vi "Module Top Level.vi"(8 "error in":errorcluster) -> (0 "error out":errorcluster)   [LabVIEW 2018, in "Testing UI 2.lvlib"]
doc: "This is the top level VI for this module. It uses a queue for communications and is stopped user a user event. The general architecture is similar to a simple queued message handler.\n\nThe VIs associated with this module are organized in a LabVIEW Library."
uses:
  Testing UI 2.lvlib
  Top Level/Shared Controls/All Data Cluster.ctl
  Top Level/Shared Controls/Acq Data.ctl
  Private Controls/UI  2 Data.ctl
  Private Controls/Module Data.ctl
  Private Controls/Module Action.ctl
  Top Level/Shared Controls/Range Updater.ctl
  Top Level/Shared Controls/APU Setup File.ctl
  Globals/Host Globals.vi
  Error Handler/Error Handler.lvlib
panel:
  in  "ARINC":bool
  in  "Main":bool
  in  "Calculated":bool
  in  "Accel Test":bool
  in  "EICAS":bool
  in  "Calibration":bool
  in  "Tab Control":T1(tab)
  out "TEUG4":dbl format="%.1f F"
  out "TUEG3":dbl format="%.1f F"
  out "TUEG2":dbl format="%.1f F"
  out "TUEG1":dbl format="%.1f F"
  out "TPO8":dbl format="%.1f F"
  out "TPO7":dbl format="%.1f F"
  out "TPO6":dbl format="%.1f F"
  out "TPO5":dbl format="%.1f F"
  out "TPO4":dbl format="%.1f F"
  out "TPO3":dbl format="%.1f F"
  out "TPO2":dbl format="%.1f F"
  out "TPO1":dbl format="%.1f F"
  out "TBAD4":dbl format="%.1f F"
  out "TBAD3":dbl format="%.1f F"
  out "TBAD2":dbl format="%.1f F"
  out "TBAD1":dbl format="%.1f F"
  out "TPI16":dbl format="%.1f F"
  out "TPI15":dbl format="%.1f F"
  out "TPI14":dbl format="%.1f F"
  out "TPI13":dbl format="%.1f F"
  out "TPI12":dbl format="%.1f F"
  out "TPI11":dbl format="%.1f F"
  out "TPI10":dbl format="%.1f F"
  out "TPI9":dbl format="%.1f F"
  out "TPI8":dbl format="%.1f F"
  out "TPI7":dbl format="%.1f F"
  out "TPI6":dbl format="%.1f F"
  out "TPI5":dbl format="%.1f F"
  out "TPI4":dbl format="%.1f F"
  out "TPI3":dbl format="%.1f F"
  out "TPI2":dbl format="%.1f F"
  out "TPI1":dbl format="%.1f F"
  out "00.00.9220.07":dbl(knob) caption="PAG-LO" scale=-50.0..150.0
  in  "00.00.9220.07":string
  out "C.38":dbl caption="TUEG Low" format="%.1f F"
  out "C.37":dbl caption="TUEG Up" format="%.1f F"
  out "C.12":cluster{dbl, dbl, dbl, dbl}(slide)={0.0, 380.23952095808386, 305.38922155688624, 392.21556886227546} caption="TEGTAVG" scale=400.0..1900.0
  out "C.12":dbl(slide) scale=400.0..1900.0
  in  "C.12":string
  out "C.25":cluster{dbl, dbl, dbl, dbl}(slide)={0.0, 380.23952095808386, 305.38922155688624, 392.21556886227546} caption="TEGT corr" scale=400.0..1900.0
  out "C.25":dbl(slide) scale=400.0..1900.0
  in  "C.25":string
  out "C.11":cluster{dbl, dbl, dbl, dbl}(slide)={0.0, 380.23952095808386, 305.38922155688624, 392.21556886227546} caption="TT1AVG" scale=0.0..150.0
  out "C.11":dbl(slide) scale=0.0..150.0
  in  "C.11":string
  out "C.02":cluster{dbl, dbl, dbl, dbl}(slide)={0.0, 380.23952095808386, 305.38922155688624, 392.21556886227546} caption="TEGT Meas" scale=400.0..1900.0
  out "C.02":dbl(slide) scale=400.0..1900.0
  in  "C.02":string
  out "C.32":dbl format="%.2f"
  out "C.31":dbl format="%.2f"
  out "00.03.9402":cluster{dbl, dbl}(knob)={0.0, 5.1101000456314445} caption="N1" scale=0.0..40640.0 scale format="%#.2f"
  out "C.17":dbl caption="MDOT" format="%.1f"
  out "C.18":dbl caption="Theta B" format="%.1f"
  out "C.19":dbl caption="PBmeas" format="%.1f"
  out "C.20":dbl caption="PBCOR" format="%.1f"
  out "C.21":dbl caption="Delta B" format="%.1f"
  out "C.22":dbl caption="Delta PAMB" format="%.1f"
  out "02.03.9227.00":dbl(knob) caption="SVTMC" scale=0.0..120.0
  out "C.29":dbl caption="HPkw" format="%.1f"
  out "02.04.9871.12":dbl caption="TkVA" format="%.1f"
  out "02.04.9871.13":dbl caption="Freq" format="%.1f"
  out "C.51":cluster{dbl, dbl, dbl, dbl}(slide)={0.0, 380.23952095808386, 305.38922155688624, 392.21556886227546} caption="Tamb" scale=55.0..125.0
  out "C.51":dbl(slide) caption="DCF" scale=55.0..125.0
  in  "C.51":string
  in  "01.01.9213.12":string
  in  "01.01.9213.13":string
  in  "01.01.9213.14":string
  in  "01.01.9213.15":string
  in  "01.01.9213.00":string
  in  "01.01.9213.01":string
  in  "01.01.9213.02":string
  in  "01.01.9213.03":string
  out "00.00.9220.12":dbl(knob) caption="PBA660" scale=0.0..50.0
  in  "00.00.9220.12":string
  out "00.00.9220.14":dbl(knob) caption="PBA290" scale=0.0..50.0
  in  "00.00.9220.14":string
  out "00.00.9220.15":dbl(knob) caption="PBA300" scale=0.0..50.0
  in  "00.00.9220.15":string
  out "00.00.9220.11":dbl(knob) caption="PES" scale=-50.0..150.0
  in  "00.00.9220.11":string
  out "00.00.9220.02":dbl(knob) caption="PFI" scale=0.0..100.0
  in  "00.00.9220.02":string
  out "00.00.9220.01":dbl(knob) caption="PFPD" scale=0.0..600.0
  in  "00.00.9220.01":string
  out "00.00.9220.03":dbl(knob) caption="POPD" scale=0.0..200.0
  in  "00.00.9220.03":string
  out "00.00.9220.08":dbl(knob) caption="PAG-HI" scale=-30.0..15.0
  in  "00.00.9220.08":string
  out "00.00.9220.09":dbl(knob) caption="PTBC" scale=-50.0..150.0
  in  "00.00.9220.09":string
  out "C.52":dbl(knob) caption="PBAD" scale=0.0..120.0
  in  "C.52":string
  out "C.49":cluster{dbl, dbl}(knob)={0.0, 94.00905280256501} caption="WBmeas"
  in  "C.49":string
  out "01.00.9213.11":cluster{dbl, dbl, dbl, dbl}(slide)={0.0, 380.23952095808386, 305.38922155688624, 392.21556886227546} caption="Tamb" scale=0.0..150.0 scale format="%.2f F"
  out "01.00.9213.11":dbl(slide) caption="TAMB" scale=0.0..150.0
  in  "01.00.9213.11":string
  out "00.00.9220.04":cluster{dbl, dbl, dbl, dbl}(slide)={0.0, 380.23952095808386, 305.38922155688624, 392.21556886227546} caption="Tamb" scale=0.0..31.0 scale format="%.2f"
  out "00.00.9220.04":dbl(slide) caption="PBAR" scale=0.0..31.0
  in  "00.00.9220.04":string
  out "C.53":cluster{dbl, dbl, dbl, dbl}(slide)={0.0, 380.23952095808386, 305.38922155688624, 392.21556886227546} caption="Tamb" scale=0.0..100.0
  out "C.53":dbl(slide) caption="POI" scale=0.0..100.0
  in  "C.53":string
  out "00.00.9220.06":cluster{dbl, dbl, dbl, dbl}(slide)={0.0, 380.23952095808386, 305.38922155688624, 392.21556886227546} caption="Tamb" scale=0.0..300.0 scale format="%.2f"
  out "00.00.9220.06":dbl(slide) caption="POD" scale=0.0..300.0
  in  "00.00.9220.06":string
  out "01.00.9213.04":cluster{dbl, dbl, dbl, dbl}(slide)={0.0, 380.23952095808386, 305.38922155688624, 392.21556886227546} caption="Tamb" scale=0.0..600.0 scale format="%.1f F"
  out "01.00.9213.04":dbl(slide) caption="TOI" scale=0.0..600.0
  in  "01.00.9213.04":string
  out "01.00.9213.07":cluster{dbl, dbl, dbl, dbl}(slide)={0.0, 380.23952095808386, 305.38922155688624, 392.21556886227546} caption="TFPI" scale=0.0..150.0
  out "01.00.9213.07":dbl(slide) scale=0.0..150.0
  out "01.00.9213.10":cluster{dbl, dbl, dbl, dbl}(slide)={0.0, 380.23952095808386, 305.38922155688624, 392.21556886227546} caption="TFC" scale=0.0..200.0
  out "01.00.9213.10":dbl(slide) scale=0.0..200.0
  in  "01.00.9213.10":string
  out "01.00.9213.02":cluster{dbl, dbl, dbl, dbl}(slide)={0.0, 380.23952095808386, 305.38922155688624, 392.21556886227546} caption="TOPD" scale=0.0..300.0
  out "01.00.9213.02":dbl(slide) scale=0.0..300.0
  out "01.00.9213.09":cluster{dbl, dbl, dbl, dbl}(slide)={0.0, 380.23952095808386, 305.38922155688624, 392.21556886227546} caption="TFFT" scale=0.0..200.0
  out "01.00.9213.09":dbl(slide) scale=0.0..200.0
  out "01.00.9213.08":cluster{dbl, dbl, dbl, dbl}(slide)={0.0, 380.23952095808386, 305.38922155688624, 392.21556886227546} caption="TLCI" scale=0.0..150.0
  out "01.00.9213.08":dbl(slide) scale=0.0..150.0
  out "01.00.9213.06":cluster{dbl, dbl, dbl, dbl}(slide)={0.0, 380.23952095808386, 305.38922155688624, 392.21556886227546} caption="TCD" scale=0.0..600.0
  out "01.00.9213.06":dbl(slide) scale=0.0..600.0
  out "TUEG Delta":dbl caption="Delta" format="%.1f F"
  out "02.04.9871.00":dbl caption="L1V" format="%.1f"
  out "02.04.9871.01":dbl caption="L2V" format="%.1f"
  out "02.04.9871.02":dbl caption="L3V" format="%.1f"
  out "02.04.9871.09":dbl caption="L1A" format="%.1f"
  out "02.04.9871.10":dbl caption="L2A" format="%.1f"
  out "02.04.9871.11":dbl caption="L3A" format="%.1f"
  out "02.04.9871.03":dbl caption="L2L1V" format="%.1f"
  out "02.04.9871.04":dbl caption="L3L2V" format="%.1f"
  out "02.04.9871.05":dbl caption="L1L3V" format="%.1f"
  out "02.04.9871.06":dbl caption="L1NV" format="%.1f"
  out "02.04.9871.07":dbl caption="L2NV" format="%.1f"
  out "02.04.9871.08":dbl caption="L3NV" format="%.1f"
  out "02.04.9871.14":dbl caption="Power" format="%.1f"
  out "RH":dbl(slide)
  in  "RH":string
  in  "02.02.9402":string
  in  "01.01.9213.07":string
  in  "01.01.9213.06":string
  in  "01.01.9213.05":string
  in  "01.01.9213.04":string
  in  "01.01.9213.11":string
  in  "01.01.9213.10":string
  in  "01.01.9213.09":string
  in  "01.01.9213.08":string
  out "C.30":cluster{dbl, dbl, dbl, dbl}(slide)={0.0, 380.23952095808386, 305.38922155688624, 392.21556886227546} caption="TBmeas" scale=0.0..600.0
  out "C.30":dbl(slide) scale=0.0..600.0
  in  "C.30":string
  out "00.00.9220.03":dbl caption="POPD"
  out "C.02":dbl caption="TEGT Meas"
  out "EGT Measured and Oil Pressure":T2(graph)
  out "C.32":dbl caption="N2 %" format="%.1f %"
  out "C.31":dbl caption="N1 %" format="%.1f %"
  out "00.03.9402":cluster{dbl, dbl}(knob)={0.0, 5.1101000456314445} scale=0.0..40400.0
  out "C.39":dbl caption="OrifDia"
  out "C.26":dbl caption="K"
  out "C.01":dbl caption="SG60"
  out "C.00":dbl caption="AIN" format="%#_g ft^2"
  out "02.03.9227.02":dbl(knob) caption="EICAS EGT" scale=0.0..2000.0
  out "02.03.9227.01":dbl(knob) caption="ECU N2" scale=0.0..40400.0
  out "CaliData":T3 caption="All Data Cluster"
  out "RawData":T3 caption="All Data Cluster"
  out "ARINCValues":string[](array[string])
  out "ARINCLabels":string[][](array[string])
  # "Enviromental Conditions"
  # "Cell Orifice Conditions"
  # "APU Bleed Air"
  # "APU INLET"
  # "TC splits"
  # "Rotor Speed"
  # "APU Fluids Status"
  # "APU EXHAUST"
  # "N1"
  # "N2"
  # "N1%"
  # "N2%"
  # "APU UNIT EXHAUST"
  # "APU Buffered Air Pressures"
  # "Standard Corrections"
  # "APU MISC"
  # "BLEED"
  # "Bleed"
  # "Day"
  # "APU Temperatures"
  # "Power"
  # "Load Bank"
  # "Acceleration Test"
  # "Rotor Speed"
  # "Default:  42000       2000      100"
  # "N1"
  # "N1"
  # "Calculated"
  # "User Inputs:"
  # "A \nA = K(2*gc/R)^0.5"
  # "P1\nPOIab * 70.726"
  # "PB meas P  (PSI)\n\nPBADab*(0.491154)"
  # "HPkw\nPower *1.34102209"
  # "SGII\nSG60*(1+(0.003688+-0.006518*SG60+0.003194*SG60^2)*(60-TFFT));"
  # "PODF\nPOD * 5.2"
  # "B \nB = Y1(1-(P2/P1))0.5 ="
  # "RhoFuel\n-0.0249876*TFFT + 52.2080853"
  # "PBCOR\n((PBMEAS P) / ((Pbar*0.491154)/14.7))"
  # "P2\nP1-PODF"
  # "RhoH2O\n0.000000162*TFFT^3 - 0.000127783*TFFT^2 + 0.008195247*TFFT + 62.294045686"
  # "C \nC = (TOI)^0.5/P1*A\nTOI to Rankeine for calculation"
  # "DeltaB\n((PBMeas P))/14.7;"
  # "P1P2\nP1-P2"
  # "SGCal\nRhoFuel / RhoH2O"
  # "dPAMB\n(PBAR * 0.491154)/(14.7/))"
  # "WBmeas \n(A*B)/C"
  # "RP1P2\n(P1-P2)/P1"
  # "Rho_air\n(PSAVG *144)/ 53.35*(TPIAVG + 459.67)"
  # "Pamb P\n(PBAR*0.491154)"
  # "WBcor \nWBCOR = WBMEAS/dPAMB"
  # "VIN\n(2/Rho_air)*(PDAVG - PSAVG)^ 1/2"
  # "Y1\n\n3.025\n=-0.2991*RP1P2 + 1.0006\n\n4\n=-0.305*RP1P2 + 1.0008\n\n5\n=-0.3.18*RP1P2 + 1.001"
  # "DPPb\n[14.7*(PBMEAS P+ PBAR)/(PBAR)]-14.7"
  # "MDOT\nMDOT = Rho_air * AIN * VIN"
  # "DCF \nWBmeas*((qB)^0.5)/DeltaB"
  # "TEGTcorr\nTEGTMeas - 11 (PBCOR-PBCOR-from-table)"
  # "ThetaB\n(TBMEAS + 459.7)/518.7"
  # "FlowPPH\n= Flow(GPH)*60*RhoFuel/7.48"
  # "EICAS"
  # "Description"
  # "Units"
  # "Value"
  # "Label"
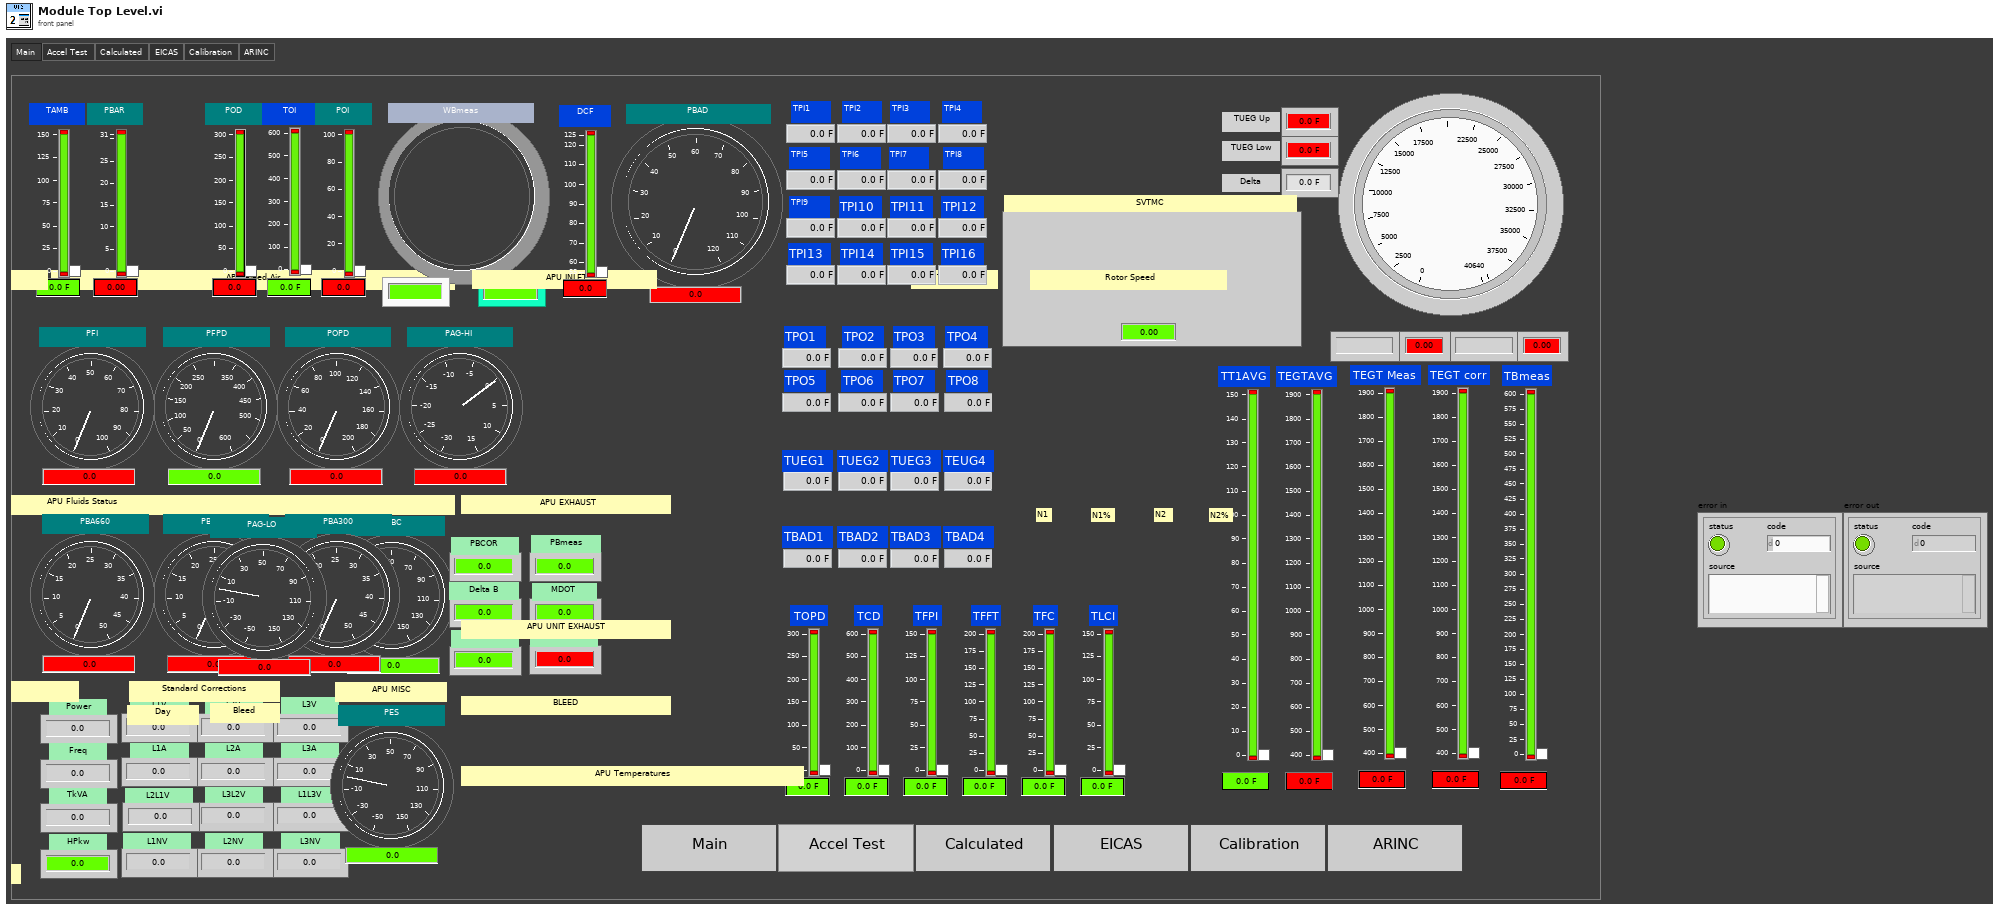
[diagram p1: front panel]
types:
  T1 = enum32{"Main", "Accel Test", "Calculated", "EICAS", "Calibration", "ARINC"}
  T2 = cluster{"RPM":dbl, "TEGT ":dbl, "Oil Pressure":dbl}
  T3 = typedef "All Data Cluster.ctl" = cluster{"AI":T4, "Accel Data":cluster{"Accel RMS(in/sec2)":dbl[], "Accel Peak(in/sec2)":dbl[], "Velocity RMS(in/sec)":dbl[], "Velocity Peak(in/sec)":dbl[]}, "Temps":cluster{"01-00-9213":dbl[], "01-01-9213":dbl[], "01-02-9213":dbl[]}, "00-03-9402(RPM)":dbl[], "02-04-9871":dbl[], "ARINC":sgl[]}
  T4 = typedef "Acq Data.ctl" = cluster{"00-00-9220":dbl[], "00-01-9220":dbl[], "02-02-9219":dbl[], "02-03-9227":dbl[], "02-05-9205":dbl[]}
  T5 = typedef "Testing UI 2.lvlib/UI  2 Data.ctl" = cluster{"[Array Of Threshold Refs]":refnum<vi>[], "[Slider Indicator Refs]":refnum<vi>[], "[Knob Indicator Refs]":refnum<vi>[], "[Digital Indicator Refs]":refnum<vi>[], "[Digital Temp]":refnum<vi>[]}
  T6 = enum32{"Main", "Accel Test", "Calculated", "EICAS", "Calibration"}
  T7 = enum32{"Invalid", "Standard", "Closed", "Hidden", "Minimized", "Maximized"}
  T8 = typedef "APU Setup File.ctl" = cluster{"Sensor Info":string[][], "Variables":string[][], "CMM Table 106":string[][], "CMM Table 106B ":string[][], "Accel Config":string[][], "Report Sheet 1":string[][], "Report Sheet 2":string[][], "Report Sheet 3":string[][]}
  T9 = typedef "Range Updater.ctl" = cluster{"[Digital Indicator Refs]":refnum<vi>[], "[Knob Indicator Refs]":refnum<vi>[], "[Slider Indicator Refs]":refnum<vi>[], "[Bool Indicator Refs]":refnum<vi>[], "[[Sensor Info]]":string[][], "[Array Of Threshold Refs]":refnum<vi>[]}
  T10 = typedef "Testing UI 2.lvlib/Module Data.ctl" = cluster{"Data":variant, "Action":T11}
  T11 = typedef "Testing UI 2.lvlib/Module Action.ctl" = enum8{"Init", "Open FP", "Error", "Exit", "Timeout", "Load APU Setup"}
  T12 = typedef "Calculated Data.ctl" = cluster{"C.00":dbl, "C.01":dbl, "C.02":dbl, "C.03":dbl, "C.04":dbl, "C.05":dbl, "C.06":dbl, "C.07":dbl, "C.08":dbl, "C.09":dbl, "C.10":dbl, "C.11":dbl, "C.12":dbl, "C.13":dbl, "C.14":dbl, "C.15":dbl, "C.16":dbl, "C.17":dbl, "C.18":dbl, "C.19":dbl, "C.20":dbl, "C.21":dbl, "C.22":dbl, "C.23":dbl, "C.24":dbl, "C.25":dbl, "C.26":dbl, "C.27":dbl, "C.28":dbl, "C.29":dbl, "C.30":dbl, "C.31":dbl, "C.32":dbl, "C.33":dbl, "C.34":dbl, "C.35":dbl, "C.36":dbl, "C.37":dbl, "C.38":dbl, "C.39":dbl, "C.40":dbl, "C.41":dbl, "C.42":dbl, "C.43":dbl, "C.44":dbl, "C.45":dbl, "C.46":dbl, "C.47":dbl, "C.48":dbl, "C.49":dbl, "C.50":dbl, "C.51":dbl, "C.52":dbl, "C.53":dbl, "C.54":dbl, "C.55":dbl, "C.56":dbl, "C.57":dbl, "C.58":dbl, "C.59":dbl, "C.60":dbl, "C.61":dbl, "C.62":dbl}
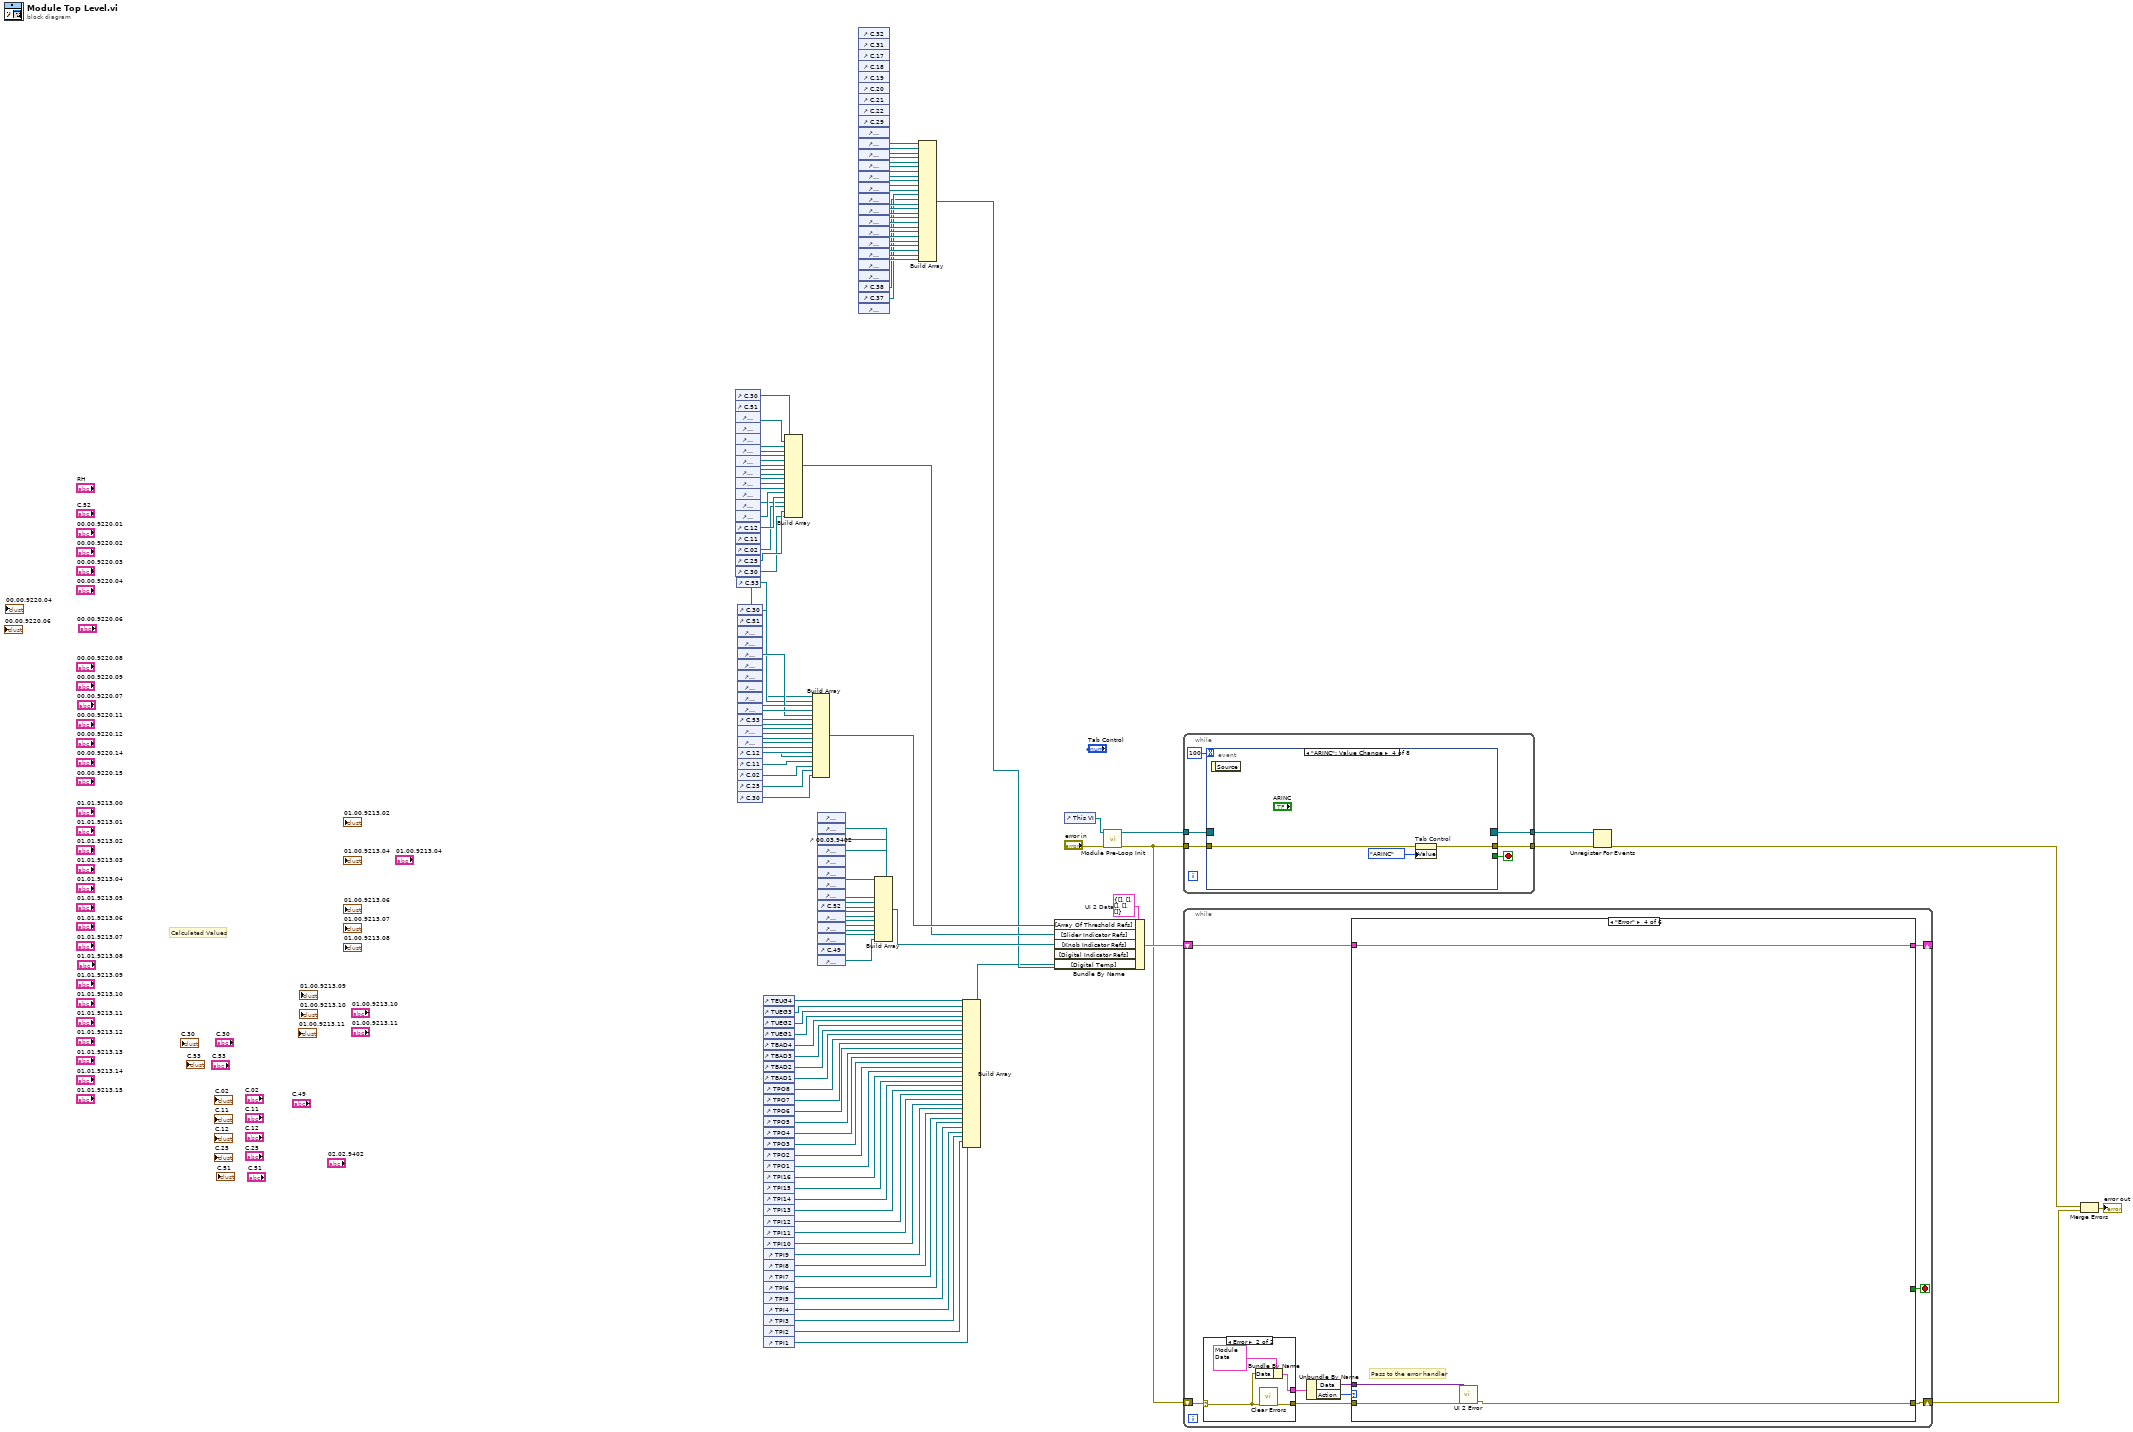
[diagram p0: block diagram]
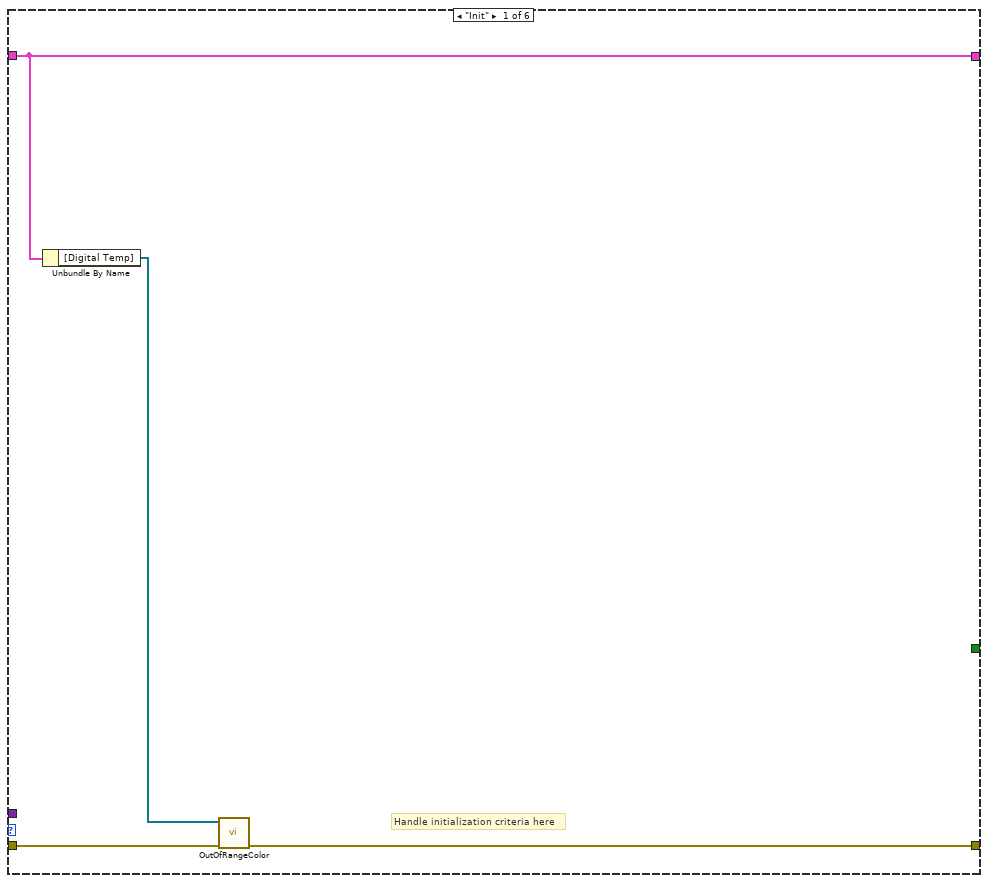
[diagram p2: hidden frame]
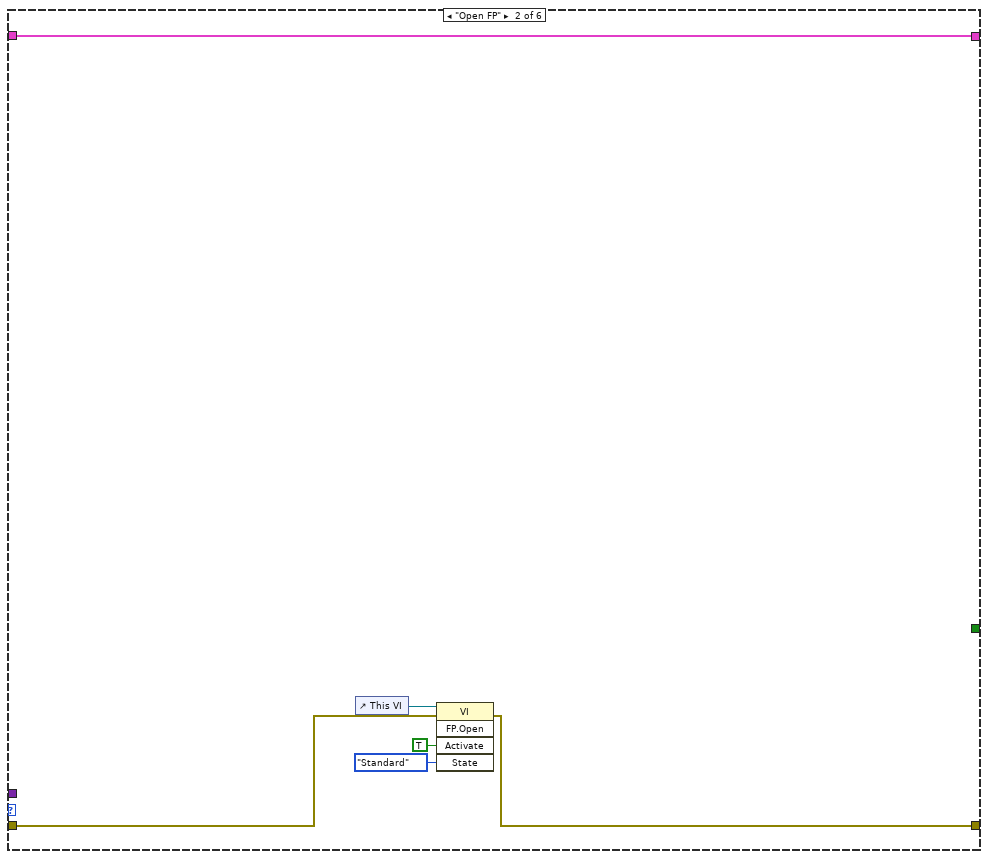
[diagram p3: hidden frame]
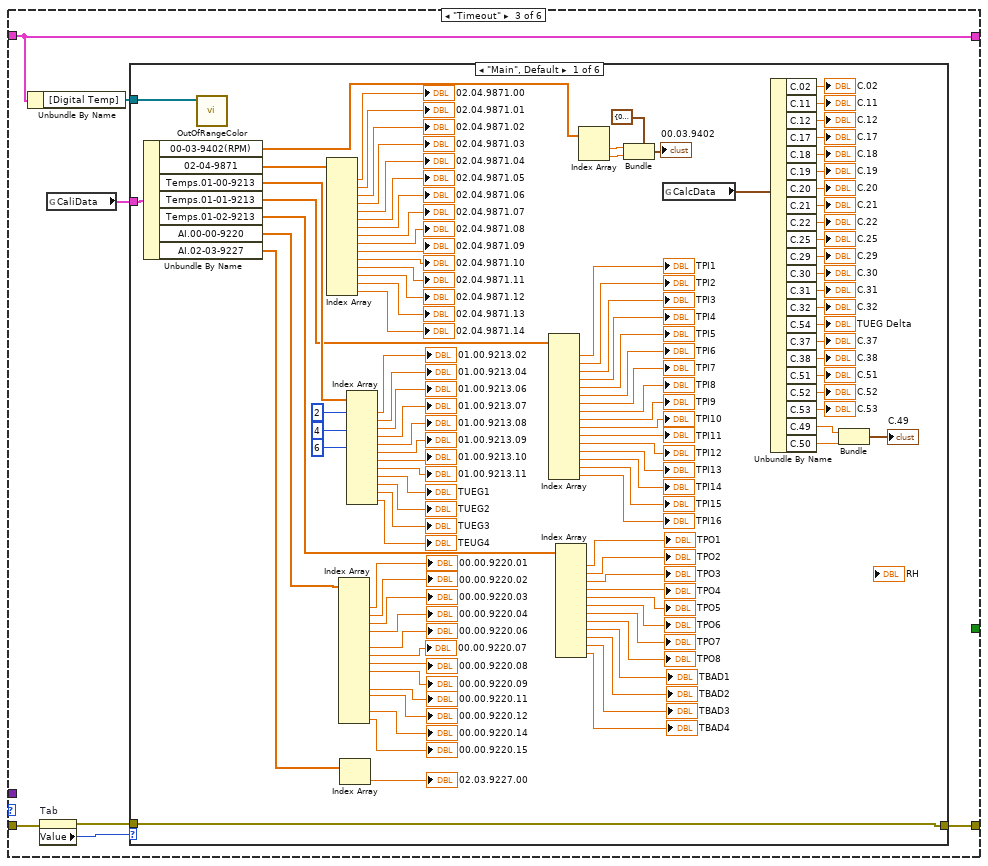
[diagram p4: hidden frame]
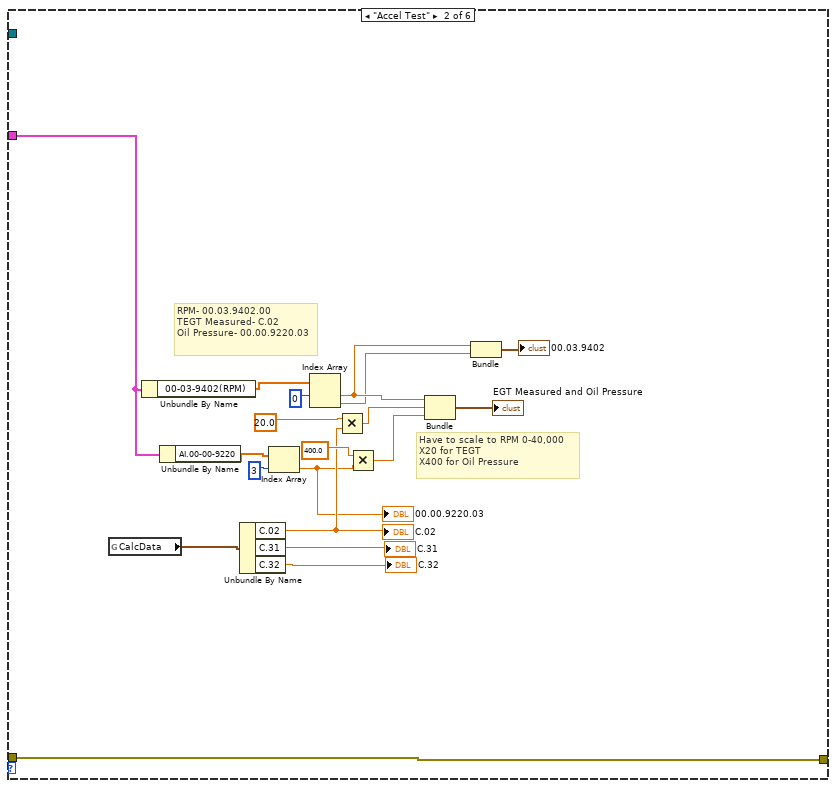
[diagram p5: hidden frame]
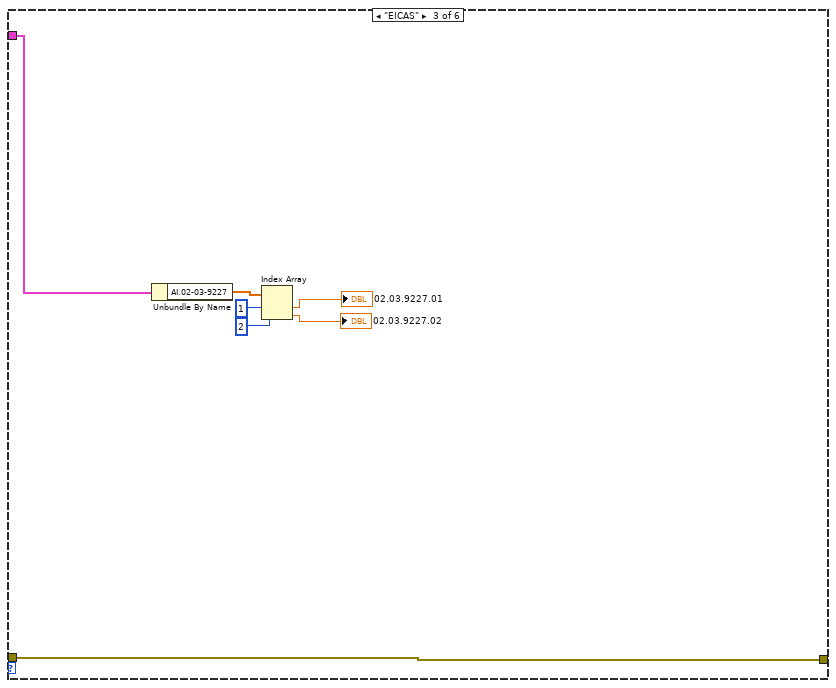
[diagram p6: hidden frame]
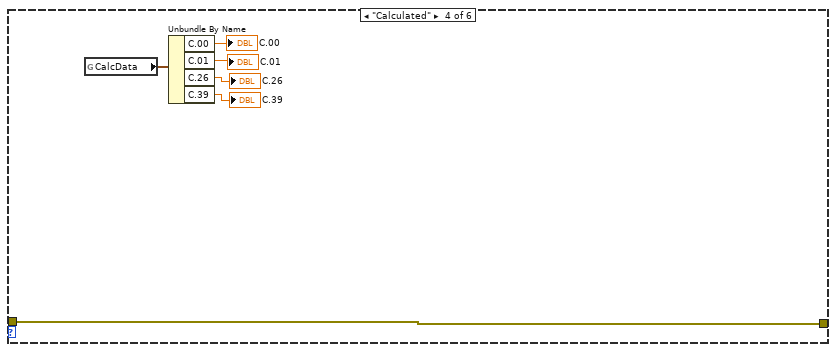
[diagram p7: hidden frame]
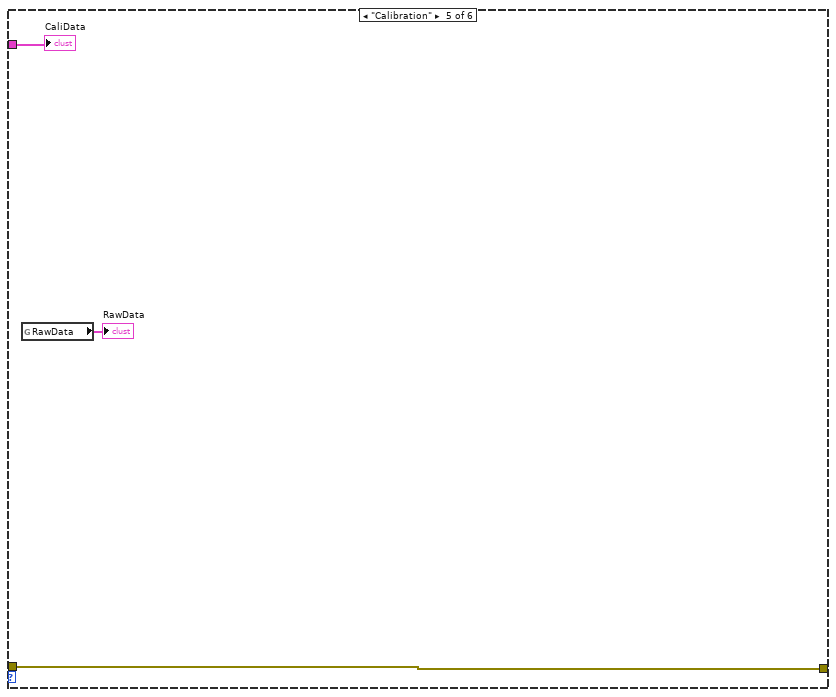
[diagram p8: hidden frame]
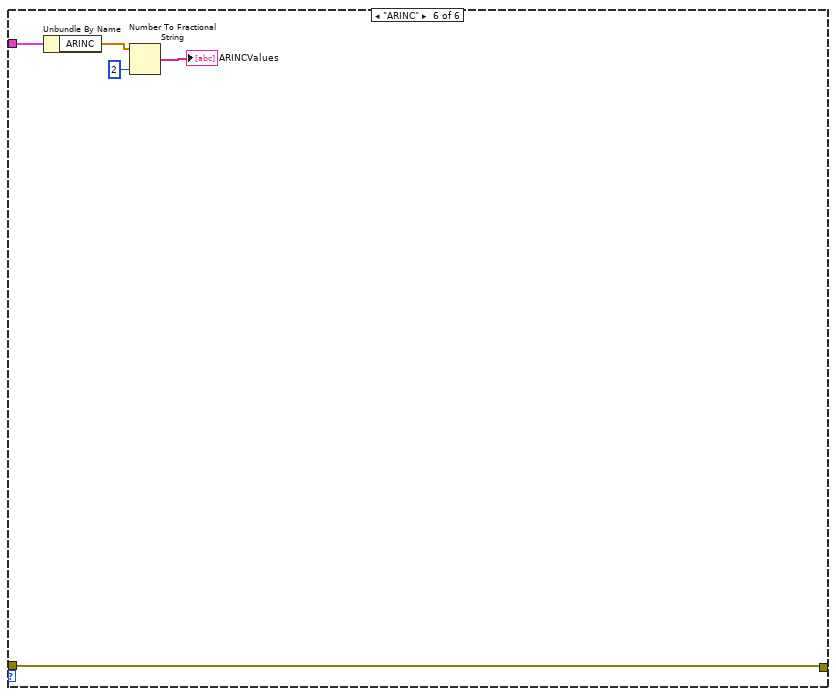
[diagram p9: hidden frame]
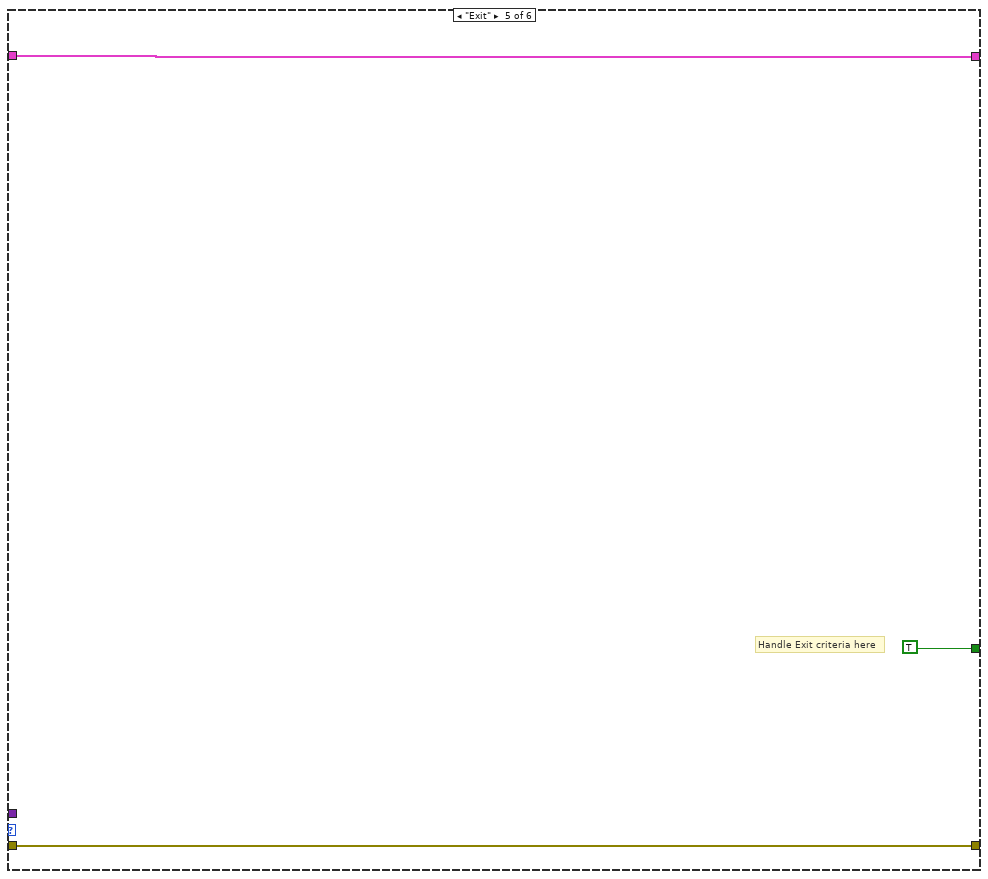
[diagram p10: hidden frame]
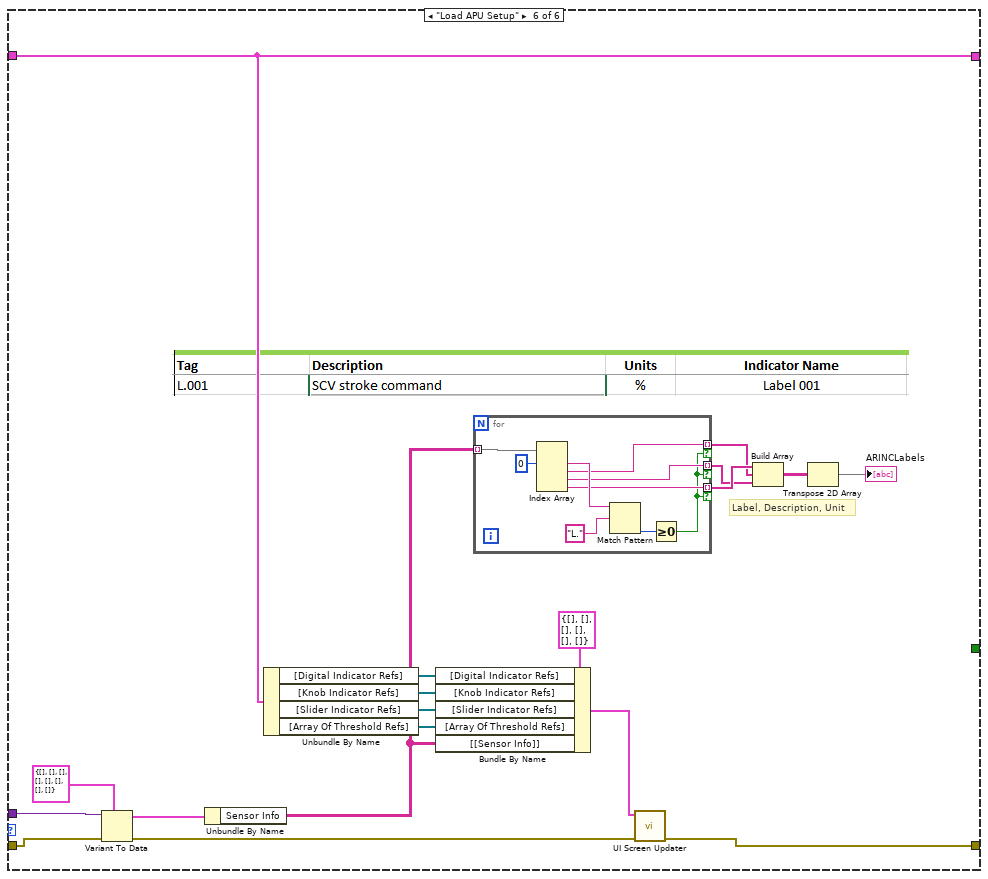
[diagram p11: hidden frame]
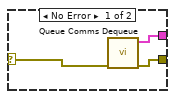
[diagram p12: hidden frame]
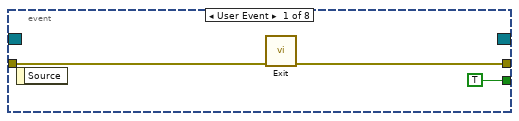
[diagram p13: hidden frame]
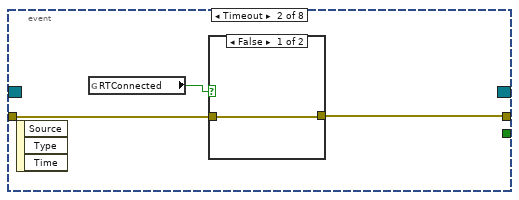
[diagram p14: hidden frame]
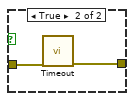
[diagram p15: hidden frame]
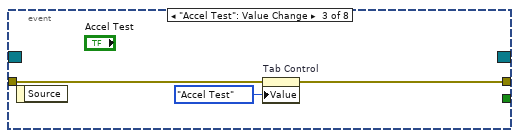
[diagram p16: hidden frame]
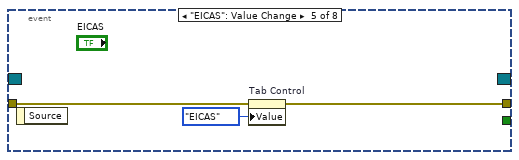
[diagram p17: hidden frame]
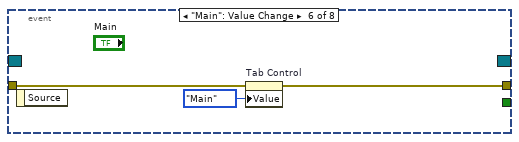
[diagram p18: hidden frame]
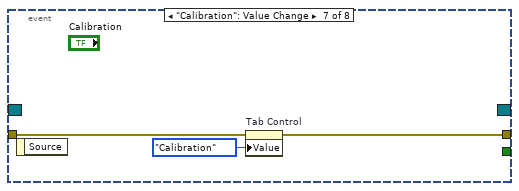
[diagram p19: hidden frame]
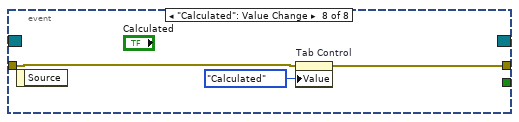
[diagram p20: hidden frame]
diagram:
  w116 = T5 {"[Array Of Threshold Refs]"=[], "[Slider Indicator Refs]"=[], "[Knob Indicator Refs]"=[], "[Digital Indicator Refs]"=[], "[Digital Temp]"=[]}  # UI 2 Data
  # "Calculated Values"
  n1 = control-ref of="C.30"() -> (w37:refnum<vi>)
  n2 = control-ref of="C.51"() -> (w38:refnum<vi>)
  n3 = control-ref of="01.00.9213.06"() -> (w102:refnum<vi>)
  n4 = control-ref of="01.00.9213.08"() -> (w101:refnum<vi>)
  n5 = control-ref of="01.00.9213.09"() -> (w100:refnum<vi>)
  n6 = control-ref of="01.00.9213.02"() -> (w99:refnum<vi>)
  n7 = control-ref of="01.00.9213.10"() -> (w98:refnum<vi>)
  n8 = control-ref of="01.00.9213.07"() -> (w97:refnum<vi>)
  n9 = control-ref of="01.00.9213.04"() -> (w96:refnum<vi>)
  n10 = control-ref of="00.00.9220.06"() -> (w95:refnum<vi>)
  n11 = control-ref of="00.00.9220.04"() -> (w93:refnum<vi>)
  n12 = control-ref of="01.00.9213.11"() -> (w92:refnum<vi>)
  n13 = control-ref of="C.12"() -> (w45:refnum<vi>)
  n14 = control-ref of="C.11"() -> (w44:refnum<vi>)
  n15 = control-ref of="C.02"() -> (w3:refnum<vi>)
  n16 = control-ref of="C.25"() -> (w43:refnum<vi>)
  n17 = control-ref of="C.30"() -> (w42:refnum<vi>)
  n18 = control-ref of="C.53"() -> (w94:refnum<vi>)
  n19 = control-ref of="C.30"() -> (w35:refnum<vi>)
  n20 = control-ref of="C.51"() -> (w36:refnum<vi>)
  n21 = control-ref of="01.00.9213.06"() -> (w114:refnum<vi>)
  n22 = control-ref of="01.00.9213.08"() -> (w113:refnum<vi>)
  n23 = control-ref of="01.00.9213.09"() -> (w112:refnum<vi>)
  n24 = control-ref of="01.00.9213.02"() -> (w111:refnum<vi>)
  n25 = control-ref of="01.00.9213.10"() -> (w110:refnum<vi>)
  n26 = control-ref of="01.00.9213.07"() -> (w109:refnum<vi>)
  n27 = control-ref of="01.00.9213.04"() -> (w108:refnum<vi>)
  n28 = control-ref of="00.00.9220.06"() -> (w107:refnum<vi>)
  n29 = control-ref of="C.53"() -> (w106:refnum<vi>)
  n30 = control-ref of="00.00.9220.04"() -> (w105:refnum<vi>)
  n31 = control-ref of="01.00.9213.11"() -> (w104:refnum<vi>)
  n32 = control-ref of="C.12"() -> (w50:refnum<vi>)
  n33 = control-ref of="C.11"() -> (w49:refnum<vi>)
  n34 = control-ref of="C.02"() -> (w48:refnum<vi>)
  n35 = control-ref of="C.25"() -> (w47:refnum<vi>)
  n36 = control-ref of="C.30"() -> (w46:refnum<vi>)
  n37 = control-ref of="TEUG4"() -> (w34:refnum<vi>)
  n38 = control-ref of="TUEG3"() -> (w33:refnum<vi>)
  n39 = control-ref of="TUEG2"() -> (w32:refnum<vi>)
  n40 = control-ref of="TUEG1"() -> (w31:refnum<vi>)
  n41 = control-ref of="TBAD4"() -> (w30:refnum<vi>)
  n42 = control-ref of="TBAD3"() -> (w29:refnum<vi>)
  n43 = control-ref of="TBAD2"() -> (w28:refnum<vi>)
  n44 = control-ref of="TBAD1"() -> (w27:refnum<vi>)
  n45 = control-ref of="TPO8"() -> (w26:refnum<vi>)
  n46 = control-ref of="TPO7"() -> (w25:refnum<vi>)
  n47 = control-ref of="TPO6"() -> (w24:refnum<vi>)
  n48 = control-ref of="TPO5"() -> (w23:refnum<vi>)
  n49 = control-ref of="TPO4"() -> (w22:refnum<vi>)
  n50 = control-ref of="TPO3"() -> (w21:refnum<vi>)
  n51 = control-ref of="TPO2"() -> (w20:refnum<vi>)
  n52 = control-ref of="TPO1"() -> (w19:refnum<vi>)
  n53 = control-ref of="TPI16"() -> (w18:refnum<vi>)
  n54 = control-ref of="TPI15"() -> (w17:refnum<vi>)
  n55 = control-ref of="TPI14"() -> (w16:refnum<vi>)
  n56 = control-ref of="TPI13"() -> (w15:refnum<vi>)
  n57 = control-ref of="TPI12"() -> (w14:refnum<vi>)
  n58 = control-ref of="TPI11"() -> (w13:refnum<vi>)
  n59 = control-ref of="TPI10"() -> (w12:refnum<vi>)
  n60 = control-ref of="TPI9"() -> (w11:refnum<vi>)
  n61 = control-ref of="TPI8"() -> (w10:refnum<vi>)
  n62 = control-ref of="TPI7"() -> (w9:refnum<vi>)
  n63 = control-ref of="TPI6"() -> (w8:refnum<vi>)
  n64 = control-ref of="TPI5"() -> (w7:refnum<vi>)
  n65 = control-ref of="TPI4"() -> (w6:refnum<vi>)
  n66 = control-ref of="TPI3"() -> (w5:refnum<vi>)
  n67 = control-ref of="TPI2"() -> (w4:refnum<vi>)
  n68 = control-ref of="TPI1"() -> (w2:refnum<vi>)
  n69 = Build Array(w37, w38, w102, w101, w100, w99, w98, w97, w96, w95, w94, w93, w92, w45, w44, w3, w43, w42) -> (w91:refnum<vi>[])
  n70 = Build Array(w35, w36, w114, w113, w112, w111, w110, w109, w108, w107, w106, w105, w104, w50, w49, w48, w47, w46) -> (w103:refnum<vi>[])
  n71 = control-ref of="00.00.9220.15"() -> (w90:refnum<vi>)
  n72 = control-ref of="02.03.9227.00"() -> (w89:refnum<vi>)
  n73 = control-ref of="00.03.9402"() -> (w88:refnum<vi>)
  n74 = control-ref of="00.00.9220.12"() -> (w87:refnum<vi>)
  n75 = control-ref of="00.00.9220.01"() -> (w86:refnum<vi>)
  n76 = control-ref of="00.00.9220.03"() -> (w85:refnum<vi>)
  n77 = control-ref of="00.00.9220.09"() -> (w84:refnum<vi>)
  n78 = control-ref of="00.00.9220.14"() -> (w83:refnum<vi>)
  n79 = control-ref of="C.52"() -> (w82:refnum<vi>)
  n80 = control-ref of="00.00.9220.11"() -> (w81:refnum<vi>)
  n81 = control-ref of="00.00.9220.02"() -> (w80:refnum<vi>)
  n82 = control-ref of="00.00.9220.08"() -> (w79:refnum<vi>)
  n83 = control-ref of="C.49"() -> (w78:refnum<vi>)
  n84 = control-ref of="00.00.9220.07"() -> (w39:refnum<vi>)
  n85 = control-ref of="C.32"() -> (w77:refnum<vi>)
  n86 = control-ref of="C.31"() -> (w76:refnum<vi>)
  n87 = control-ref of="C.17"() -> (w75:refnum<vi>)
  n88 = control-ref of="C.18"() -> (w74:refnum<vi>)
  n89 = control-ref of="C.19"() -> (w73:refnum<vi>)
  n90 = control-ref of="C.20"() -> (w72:refnum<vi>)
  n91 = control-ref of="C.21"() -> (w71:refnum<vi>)
  n92 = control-ref of="C.22"() -> (w70:refnum<vi>)
  n93 = control-ref of="C.29"() -> (w69:refnum<vi>)
  n94 = control-ref of="02.04.9871.12"() -> (w68:refnum<vi>)
  n95 = control-ref of="02.04.9871.13"() -> (w67:refnum<vi>)
  n96 = control-ref of="02.04.9871.14"() -> (w66:refnum<vi>)
  n97 = control-ref of="02.04.9871.08"() -> (w65:refnum<vi>)
  n98 = control-ref of="02.04.9871.07"() -> (w64:refnum<vi>)
  n99 = control-ref of="02.04.9871.06"() -> (w63:refnum<vi>)
  n100 = control-ref of="02.04.9871.05"() -> (w62:refnum<vi>)
  n101 = control-ref of="02.04.9871.04"() -> (w61:refnum<vi>)
  n102 = control-ref of="02.04.9871.03"() -> (w60:refnum<vi>)
  n103 = control-ref of="02.04.9871.11"() -> (w59:refnum<vi>)
  n104 = control-ref of="02.04.9871.10"() -> (w58:refnum<vi>)
  n105 = control-ref of="02.04.9871.09"() -> (w57:refnum<vi>)
  n106 = control-ref of="02.04.9871.02"() -> (w56:refnum<vi>)
  n107 = control-ref of="02.04.9871.01"() -> (w55:refnum<vi>)
  n108 = control-ref of="C.38"() -> (w40:refnum<vi>)
  n109 = control-ref of="C.37"() -> (w41:refnum<vi>)
  n110 = control-ref of="02.04.9871.00"() -> (w54:refnum<vi>)
  n111 = Build Array(w90, w89, w88, w87, w86, w85, w84, w83, w82, w81, w80, w79, w78, w39) -> (w53:refnum<vi>[])
  n112 = Build Array(w77, w76, w75, w74, w73, w72, w71, w70, w69, w68, w67, w41, w40, w66, w65, w64, w63, w62, w61, w60, w59, w58, w57, w56, w55, w54) -> (w52:refnum<vi>[])
  n113 = Build Array(w34, w33, w32, w31, w30, w29, w28, w27, w26, w25, w24, w23, w22, w21, w20, w19, w18, w17, w16, w15, w14, w13, w12, w11, w10, w9, w8, w7, w6, w5, w4, w2) -> (w1:refnum<vi>[])
  n114 = Bundle By Name(cluster=w116, "[Array Of Threshold Refs]"=w103, "[Slider Indicator Refs]"=w91, "[Knob Indicator Refs]"=w53, "[Digital Indicator Refs]"=w52, "[Digital Temp]"=w1) -> (w115:T5)
  n115 = control-ref of="This VI"() -> (w124:refnum<vi>)
  n116 = call "Module Pre-Loop Init.vi"("error in (no error)"="error in", "Top Level VI Ref in"=w124) -> ("error out"=w51:errorcluster, "User Event Stop Ref"=w122:refnum<event-registration>)  [unwired: 8 in]
  n117 = while {
    tunnel: w122 -> [w130]
    tunnel: [w129] -> w120
    tunnel: w51 -> [w128]
    tunnel: [w126] -> w121
    stop <- w127 stop-if-true
    n118 = event shown="[3] \"ARINC\": Value Change" {
      selector: w130 -> [_ _ _ _ _ _ _ _]
      dyn-events: [_ _ _ _ _ _ _ _] -> w126
      timeout: 100 -> [_ _ _ _ _ _ _ _]
      tunnel: [w132 w135 w141 w143 w147 w150 w153 w156] -> w129
      tunnel: w128 -> [w131 w136 w142 w145 w148 w151 w154 w157]
      tunnel: [TRUE _ _ _ _ _ _ _] -> w127
      event User Event {
        n119 = event-data() -> ()  [unwired: 1 in, 1 out]
        n120 = call "Exit.vi"("error in"=w131) -> ("error out"=w132:errorcluster)  [unwired: 10 in]
      }
      event Timeout {
        n121 = event-data() -> ()  [unwired: 1 in, 3 out]
        n122 = global read "Host Globals.vi" "RTConnected"() -> (w134:bool)
        n123 = case shown="False" w134 {
          tunnel: w136 -> [w137 w139]
          tunnel: [w137 w138] -> w135
          frame False {
          }
          frame True {
            n124 = call "Timeout.vi"("error in (no error)"=w139) -> ("error out"=w138:errorcluster)  [unwired: 10 in]
          }
        }
      }
      event "Accel Test": Value Change {
        n125 = event-data() -> ()  [unwired: 1 in, 1 out]
        n126 = property on="Tab Control" class="TabCtl (strict)"(error in=w142, "Value"=T6."Accel Test" ("Tab Control")) -> (error out=w141:errorcluster)  [unwired: 1 in, 1 out]
      }
      event "ARINC": Value Change {
        n127 = event-data() -> ()  [unwired: 1 in, 1 out]
        n128 = property on="Tab Control" class="TabCtl (strict)"(error in=w145, "Value"=T1."ARINC" ("Tab Control")) -> (error out=w143:errorcluster)  [unwired: 1 in, 1 out]
      }
      event "EICAS": Value Change {
        n129 = event-data() -> ()  [unwired: 1 in, 1 out]
        n130 = property on="Tab Control" class="TabCtl (strict)"(error in=w148, "Value"=T6."EICAS" ("Tab Control")) -> (error out=w147:errorcluster)  [unwired: 1 in, 1 out]
      }
      event "Main": Value Change {
        n131 = event-data() -> ()  [unwired: 1 in, 1 out]
        n132 = property on="Tab Control" class="TabCtl (strict)"(error in=w151, "Value"=T6."Main" ("Tab Control")) -> (error out=w150:errorcluster)  [unwired: 1 in, 1 out]
      }
      event "Calibration": Value Change {
        n133 = event-data() -> ()  [unwired: 1 in, 1 out]
        n134 = property on="Tab Control" class="TabCtl (strict)"(error in=w154, "Value"=T6."Calibration" ("Tab Control")) -> (error out=w153:errorcluster)  [unwired: 1 in, 1 out]
      }
      event "Calculated": Value Change {
        n135 = event-data() -> ()  [unwired: 1 in, 1 out]
        n136 = property on="Tab Control" class="TabCtl (strict)"(error in=w157, "Value"=T6."Calculated" ("Tab Control")) -> (error out=w156:errorcluster)  [unwired: 1 in, 1 out]
      }
    }
  }
  n137 = while {
    shift-right: [w162] -> w119
    shift-left: w51 -> [w161]
    shift-right: [w160] -> _
    shift-left: w115 -> [w159]
    stop <- w158 stop-if-true
    n138 = case shown="Error" w161 {
      selector: w161 -> [w368 w371]
      tunnel: [w369 w372] -> w166
      tunnel: [w367 w370] -> w163
      frame No Error {
        n139 = call "Queue Comms Dequeue.vi"("error in (no error)"=w368) -> ("error out"=w367:errorcluster, "element"=w369:T10)  [unwired: 9 in]
      }
      frame Error {
        n140 = Bundle By Name(cluster=T10 {"Data"=variant, "Action"=enum."Error"} ("element"), "Data"=w371) -> (w372:T10)
        n141 = call <vilib>:"Clear Errors.vi"("error in (no error)"=w371) -> ("error out"=w370:errorcluster)  [unwired: 5 in, 1 out]
      }
    }
    n142 = Unbundle By Name(w166) -> ("Data"=w164:variant, "Action"=w165:T11)
    n143 = case shown="\"Error\"" w165 {
      tunnel: w164 -> [_ _ _ w334 _ w357]
      tunnel: w163 -> [w169 w171 w181 w333 w336 w356]
      tunnel: [w169 w170 w182 w332 w336 w353] -> w162
      tunnel: [_ _ _ _ TRUE _] -> w158
      tunnel: [w168 w175 w177 w335 w337 w355] -> w160
      tunnel: w159 -> [w168 w175 w177 w335 w337 w355]
      frame "Init" {
        # "Handle initialization criteria here"
        n144 = Unbundle By Name(w168) -> ("[Digital Temp]"=w167:refnum<vi>[])
        n145 = call "OutOfRangeColor.vi"("Array"=w167) -> ()  [unwired: 11 in]
      }
      frame "Open FP" {
        n146 = control-ref of="This VI"() -> (w174:refnum<vi>)
        n147 = invoke class="VI" method="FP.Open"(reference=w174, error in=w171, "Activate"=TRUE ("Activate?"), "State"=T7."Standard") -> (error out=w170:errorcluster)  [unwired: 1 in, 4 out]
      }
      frame "Timeout" {
        n148 = Unbundle By Name(w177) -> ("[Digital Temp]"=w176:refnum<vi>[])
        n149 = property on="Tab" class="TabCtl (strict)"(error in=w181) -> (error out=w180:errorcluster, "Value"=w179:T1)  [unwired: 1 in, 1 out]
        n150 = global read "Host Globals.vi" "CaliData"() -> (w178:T3)
        n151 = case shown="\"Main\", Default" w179 {
          tunnel: [w236 w293 w312 w318 w326 w330] -> w182
          tunnel: w180 -> [w236 w293 w312 w318 w326 w330]
          tunnel: w178 -> [w242 w292 w311 _ w324 w331]
          tunnel: w176 -> [w183 _ _ _ _ _]
          frame "Main", Default {
            n152 = Unbundle By Name(w242) -> ("00-03-9402(RPM)"=w240:dbl[], "02-04-9871"=w291:dbl[], "Temps.01-00-9213"=w254:dbl[], "Temps.01-01-9213"=w241:dbl[], "Temps.01-02-9213"=w235:dbl[], "AI.00-00-9220"=w234:dbl[], "AI.02-03-9227"=w232:dbl[])
            n153 = call "OutOfRangeColor.vi"("Array"=w183) -> ()  [unwired: 11 in]
            n154 = Index Array(array=w291) -> (element #1=→"02.04.9871.00":dbl, element #2=→"02.04.9871.01":dbl, element #3=→"02.04.9871.02":dbl, element #4=→"02.04.9871.03":dbl, element #5=→"02.04.9871.04":dbl, element #6=→"02.04.9871.05":dbl, element #7=→"02.04.9871.06":dbl, element #8=→"02.04.9871.07":dbl, element #9=→"02.04.9871.08":dbl, element #10=→"02.04.9871.09":dbl, element #11=→"02.04.9871.10":dbl, element #12=→"02.04.9871.11":dbl, element #13=→"02.04.9871.12":dbl, element #14=→"02.04.9871.13":dbl, element #15=→"02.04.9871.14":dbl)  [unwired: 15 in]
            n155 = Index Array(array=w234) -> (element #2=→"00.00.9220.01":dbl, element #3=→"00.00.9220.02":dbl, element #4=→"00.00.9220.03":dbl, element #5=→"00.00.9220.04":dbl, element #7=→"00.00.9220.06":dbl, element #8=→"00.00.9220.07":dbl, element #9=→"00.00.9220.08":dbl, element #10=→"00.00.9220.09":dbl, element #12=→"00.00.9220.11":dbl, element #13=→"00.00.9220.12":dbl, element #15=→"00.00.9220.14":dbl, element #16=→"00.00.9220.15":dbl)  [unwired: 16 in, 4 out]
            n156 = Index Array(array=w232) -> (element=→"02.03.9227.00":dbl)  [unwired: 1 in]
            n157 = Index Array(array=w254, index #1=2 ("index"), index #2=4 ("index"), index #3=6 ("index")) -> (element #1=→"01.00.9213.02":dbl, element #2=→"01.00.9213.04":dbl, element #3=→"01.00.9213.06":dbl, element #4=→"01.00.9213.07":dbl, element #5=→"01.00.9213.08":dbl, element #6=→"01.00.9213.09":dbl, element #7=→"01.00.9213.10":dbl, element #8=→"01.00.9213.11":dbl, element #9=→"TUEG1":dbl, element #10=→"TUEG2":dbl, element #11=→"TUEG3":dbl, element #12=→"TEUG4":dbl)  [unwired: 9 in]
            n158 = Index Array(array=w241) -> (element #1=→"TPI1":dbl, element #2=→"TPI2":dbl, element #3=→"TPI3":dbl, element #4=→"TPI4":dbl, element #5=→"TPI5":dbl, element #6=→"TPI6":dbl, element #7=→"TPI7":dbl, element #8=→"TPI8":dbl, element #9=→"TPI9":dbl, element #10=→"TPI10":dbl, element #11=→"TPI11":dbl, element #12=→"TPI12":dbl, element #13=→"TPI13":dbl, element #14=→"TPI14":dbl, element #15=→"TPI15":dbl, element #16=→"TPI16":dbl)  [unwired: 16 in]
            n159 = Index Array(array=w235) -> (element #1=→"TPO1":dbl, element #2=→"TPO2":dbl, element #3=→"TPO3":dbl, element #4=→"TPO4":dbl, element #5=→"TPO5":dbl, element #6=→"TPO6":dbl, element #7=→"TPO7":dbl, element #8=→"TPO8":dbl, element #9=→"TBAD1":dbl, element #10=→"TBAD2":dbl, element #11=→"TBAD3":dbl, element #12=→"TBAD4":dbl)  [unwired: 12 in]
            n160 = Index Array(array=w240) -> (element #1=w239:dbl, element #2=w237:dbl)  [unwired: 2 in]
            n161 = Bundle(cluster=cluster{"Numeric":dbl, "Numeric":dbl} {"Numeric"=0.0, "Numeric"=0.0}, "Numeric"=w239, "Numeric"=w237) -> (→"00.03.9402":cluster{"Numeric":dbl, "Numeric":dbl})
            n162 = global read "Host Globals.vi" "CalcData"() -> (w275:T12)
            n163 = Unbundle By Name(w275) -> ("C.02"=→"C.02":dbl, "C.11"=→"C.11":dbl, "C.12"=→"C.12":dbl, "C.17"=→"C.17":dbl, "C.18"=→"C.18":dbl, "C.19"=→"C.19":dbl, "C.20"=→"C.20":dbl, "C.21"=→"C.21":dbl, "C.22"=→"C.22":dbl, "C.25"=→"C.25":dbl, "C.29"=→"C.29":dbl, "C.30"=→"C.30":dbl, "C.31"=→"C.31":dbl, "C.32"=→"C.32":dbl, "C.54"=→"TUEG Delta":dbl, "C.37"=→"C.37":dbl, "C.38"=→"C.38":dbl, "C.51"=→"C.51":dbl, "C.52"=→"C.52":dbl, "C.53"=→"C.53":dbl, "C.49"=w218:dbl, "C.50"=w217:dbl)
            n164 = Bundle("C.49"=w218, "C.50"=w217) -> (→"C.49":cluster{"C.49":dbl, "C.50":dbl})  [unwired: 1 in]
          }
          frame "Accel Test" {
            # "Have to scale to RPM 0-40,000\nX20 for TEGT\nX400 for Oil Pressure"
            # "RPM- 00.03.9402.00\nTEGT Measured- C.02\nOil Pressure- 00.00.9220.03"
            n165 = global read "Host Globals.vi" "CalcData"() -> (w301:T12)
            n166 = Unbundle By Name(w292) -> ("00-03-9402(RPM)"=w303:dbl[])
            n167 = Unbundle By Name(w292) -> ("AI.00-00-9220"=w302:dbl[])
            n168 = Unbundle By Name(w301) -> ("C.02"=w300:dbl, "C.31"=→"C.31":dbl, "C.32"=→"C.32":dbl)
            "C.02" <- w300
            n169 = Index Array(array=w302, index=3) -> (element=w297:dbl)
            "00.00.9220.03" <- w297
            n170 = Index Array(array=w303, index #1=0 ("index")) -> (element #1=w295:dbl, element #2=w294:dbl)  [unwired: 1 in]
            n171 = Multiply(x=20.0, y=w300) -> (x*y=w308:dbl)
            n172 = Multiply(x=400.0, y=w297) -> (x*y=w305:dbl)
            n173 = Bundle("Numeric"=w295, w308, w305) -> (→"EGT Measured and Oil Pressure":cluster{"Numeric":dbl, dbl, dbl})  [unwired: 1 in]
            n174 = Bundle("Numeric"=w295, "Numeric"=w294) -> (→"00.03.9402":cluster{"Numeric":dbl, "Numeric":dbl})  [unwired: 1 in]
          }
          frame "EICAS" {
            n175 = Unbundle By Name(w311) -> ("AI.02-03-9227"=w317:dbl[])
            n176 = Index Array(array=w317, index #1=1 ("index"), index #2=2 ("index")) -> (element #1=→"02.03.9227.01":dbl, element #2=→"02.03.9227.02":dbl)
          }
          frame "Calculated" {
            n177 = global read "Host Globals.vi" "CalcData"() -> (w323:T12)
            n178 = Unbundle By Name(w323) -> ("C.00"=→"C.00":dbl, "C.01"=→"C.01":dbl, "C.26"=→"C.26":dbl, "C.39"=→"C.39":dbl)
          }
          frame "Calibration" {
            n179 = global read "Host Globals.vi" "RawData"() -> (→"RawData":T3)
            "CaliData" <- w324
          }
          frame "ARINC" {
            n180 = Unbundle By Name(w331) -> ("ARINC"=w329:sgl[])
            n181 = Number To Fractional String(number=w329, precision (6)=i16 2) -> (F-format string=→"ARINCValues":string[])  [unwired: 2 in]
          }
        }
      }
      frame "Error" {
        # "Pass to the error handler"
        n182 = call "UI 2 Error.vi"("error in (no error)"=w333, "Data"=w334) -> ("error out"=w332:errorcluster)  [unwired: 9 in]
      }
      frame "Exit" {
        # "Handle Exit criteria here"
      }
      frame "Load APU Setup" {
        # "Label, Description, Unit"
        n183 = Variant To Data(error in=w356, type=T8 {"Sensor Info"=[], "Variables"=[], "CMM Table 106"=[], "CMM Table 106B "=[], "Accel Config"=[], "Report Sheet 1"=[], "Report Sheet 2"=[], "Report Sheet 3"=[]} ("APU Setup File"), Variant=w357) -> (data=w345:T8, error out=w354:errorcluster)
        n184 = Unbundle By Name(w345) -> ("Sensor Info"=w344:string[][])
        n185 = Unbundle By Name(w355) -> ("[Digital Indicator Refs]"=w351:refnum<vi>[], "[Knob Indicator Refs]"=w350:refnum<vi>[], "[Slider Indicator Refs]"=w349:refnum<vi>[], "[Array Of Threshold Refs]"=w348:refnum<vi>[])
        n186 = Bundle By Name(cluster=T9 {"[Digital Indicator Refs]"=[], "[Knob Indicator Refs]"=[], "[Slider Indicator Refs]"=[], "[Bool Indicator Refs]"=[], "[[Sensor Info]]"=[], "[Array Of Threshold Refs]"=[]} ("Cluster In"), "[Digital Indicator Refs]"=w351, "[Knob Indicator Refs]"=w350, "[Slider Indicator Refs]"=w349, "[Array Of Threshold Refs]"=w348, "[[Sensor Info]]"=w344) -> (w347:T9)
        n187 = for {
          tunnel: w344 -> [w366] mode=indexing
          tunnel: [w361] -> w342 mode=indexing if=w358
          tunnel: [w360] -> w341 mode=indexing if=w358
          tunnel: [w359] -> w343 mode=indexing if=w358
          n188 = Index Array(array=w366, index #1=0 ("index")) -> (element #1=w364:string, element #2=w361:string, element #3=w360:string, element #4=w359:string)  [unwired: 3 in]
          n189 = Match Pattern(string=w364, regular expression="L.") -> (offset past match=w362:i32)  [unwired: 1 in, 3 out]
          n190 = Greater Or Equal To 0?(x=w362) -> (x >= 0?=w358:bool)
        }
        n191 = call "UI Screen Updater.vi"("error in (no error)"=w354, "Range Updater Cntrl"=w347) -> ("error out"=w353:errorcluster)  [unwired: 9 in]
        n192 = Build Array(w343, w342, w341) -> (w340:string[][])
        n193 = Transpose 2D Array(2D array=w340) -> (transposed array=→"ARINCLabels":string[][])
      }
    }
  }
  n194 = Unregister For Events(event registration refnum=w121, error in=w120) -> (error out=w117:errorcluster)
  n195 = Merge Errors(w117, w119) -> (→"error out":errorcluster)
